vi "Move Stage.vi"(8 "error in (no error)":errorcluster, 9 "Y Axis":dbl, 10 "X Axis":dbl, 11 "2-Axis Stage in":refnum<class "Sync 2-Axis Stage Controller.lvclass">) -> (0 "error out":errorcluster, 3 "2-Axis Stage out":refnum<class "Sync 2-Axis Stage Controller.lvclass">)   [LabVIEW 2022 SP3, in "Sync 2-Axis Stage Controller.lvclass"]
uses:
  Sync 2-Axis Stage Controller.lvclass
  Sync 2-Axis Stage Controller.lvclass/Sync 2-Axis Stage Controller.ctl
  Axis Objects/iMotion Controller/iMotion Controller.lvclass
  <vilib>/ErrorRing/Error Ring.xnode
  <vilib>/Utility/error.llb/Error Cluster From Error Code.vi
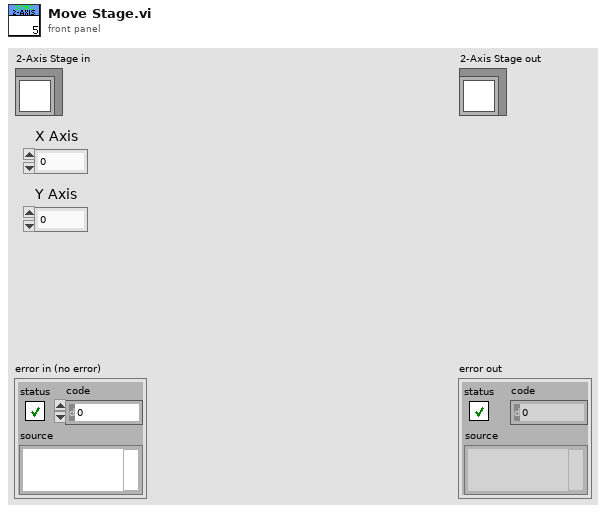
[diagram p1: front panel]
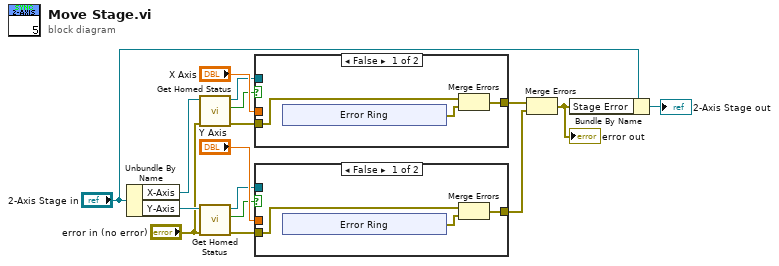
[diagram p0: block diagram]
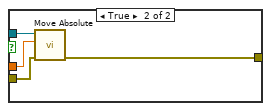
[diagram p2: hidden frame]
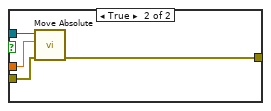
[diagram p3: hidden frame]
diagram:
  n1 = Unbundle By Name("2-Axis Stage in") -> ("X-Axis"=w9:refnum<class "iMotion Controller.lvclass">, "Y-Axis"=w8:refnum<class "iMotion Controller.lvclass">)
  n2 = call-dynamic "Get Homed Status.vi"("error in (no error)"="error in (no error)", "iMotion Controller in"=w9) -> ("error out"=w4:errorcluster, "Homed"=w1:bool, "iMotion Controller out"=w7:refnum<class "iMotion Controller.lvclass">)  [unwired: 7 in]
  n3 = call-dynamic "Get Homed Status.vi"("error in (no error)"="error in (no error)", "iMotion Controller in"=w8) -> ("error out"=w5:errorcluster, "Homed"=w2:bool, "iMotion Controller out"=w6:refnum<class "iMotion Controller.lvclass">)  [unwired: 7 in]
  n4 = case shown="False" w1 {
    tunnel: "X Axis" -> [_ w28]
    tunnel: [w18 w27] -> w13
    tunnel: w7 -> [_ w26]
    tunnel: w4 -> [w19 w25]
    frame False {
      n5 = xnode "Error Ring"() -> ("error out"=w17:errorcluster)
      n6 = Merge Errors(w19, w17) -> (w18:errorcluster)
    }
    frame True {
      n7 = call-dynamic "Move Absolute.vi"("error in (no error)"=w25, "Desired Position"=w28, "iMotion Controller in"=w26) -> ("error out"=w27:errorcluster)  [unwired: 7 in, 1 out]
    }
  }
  n8 = case shown="False" w2 {
    tunnel: "Y Axis" -> [_ w40]
    tunnel: [w30 w39] -> w12
    tunnel: w6 -> [_ w38]
    tunnel: w5 -> [w31 w37]
    frame False {
      n9 = xnode "Error Ring"() -> ("error out"=w29:errorcluster)
      n10 = Merge Errors(w31, w29) -> (w30:errorcluster)
    }
    frame True {
      n11 = call-dynamic "Move Absolute.vi"("error in (no error)"=w37, "Desired Position"=w40, "iMotion Controller in"=w38) -> ("error out"=w39:errorcluster)  [unwired: 7 in, 1 out]
    }
  }
  n12 = Merge Errors(w13, w12) -> (w10:errorcluster)
  "error out" <- w10
  n13 = Bundle By Name(cluster="2-Axis Stage in", "Stage Error"=w10) -> (→"2-Axis Stage out":refnum<class "Sync 2-Axis Stage Controller.lvclass">)
